vi "Untitled 1.vi"() -> ()   [LabVIEW 2014]
panel:
  out "Waveform Chart 2":dynamicdata(graph)
  in  "Result":dbl
  out "Waveform Chart":dbl(graph)
  in  "Hf":dbl
  out "Elapsed Time (s)":dbl
  in  "H0":dbl
  out "Numeric":dbl
  out "Tank":dbl(slide) scale=0.0..0.3
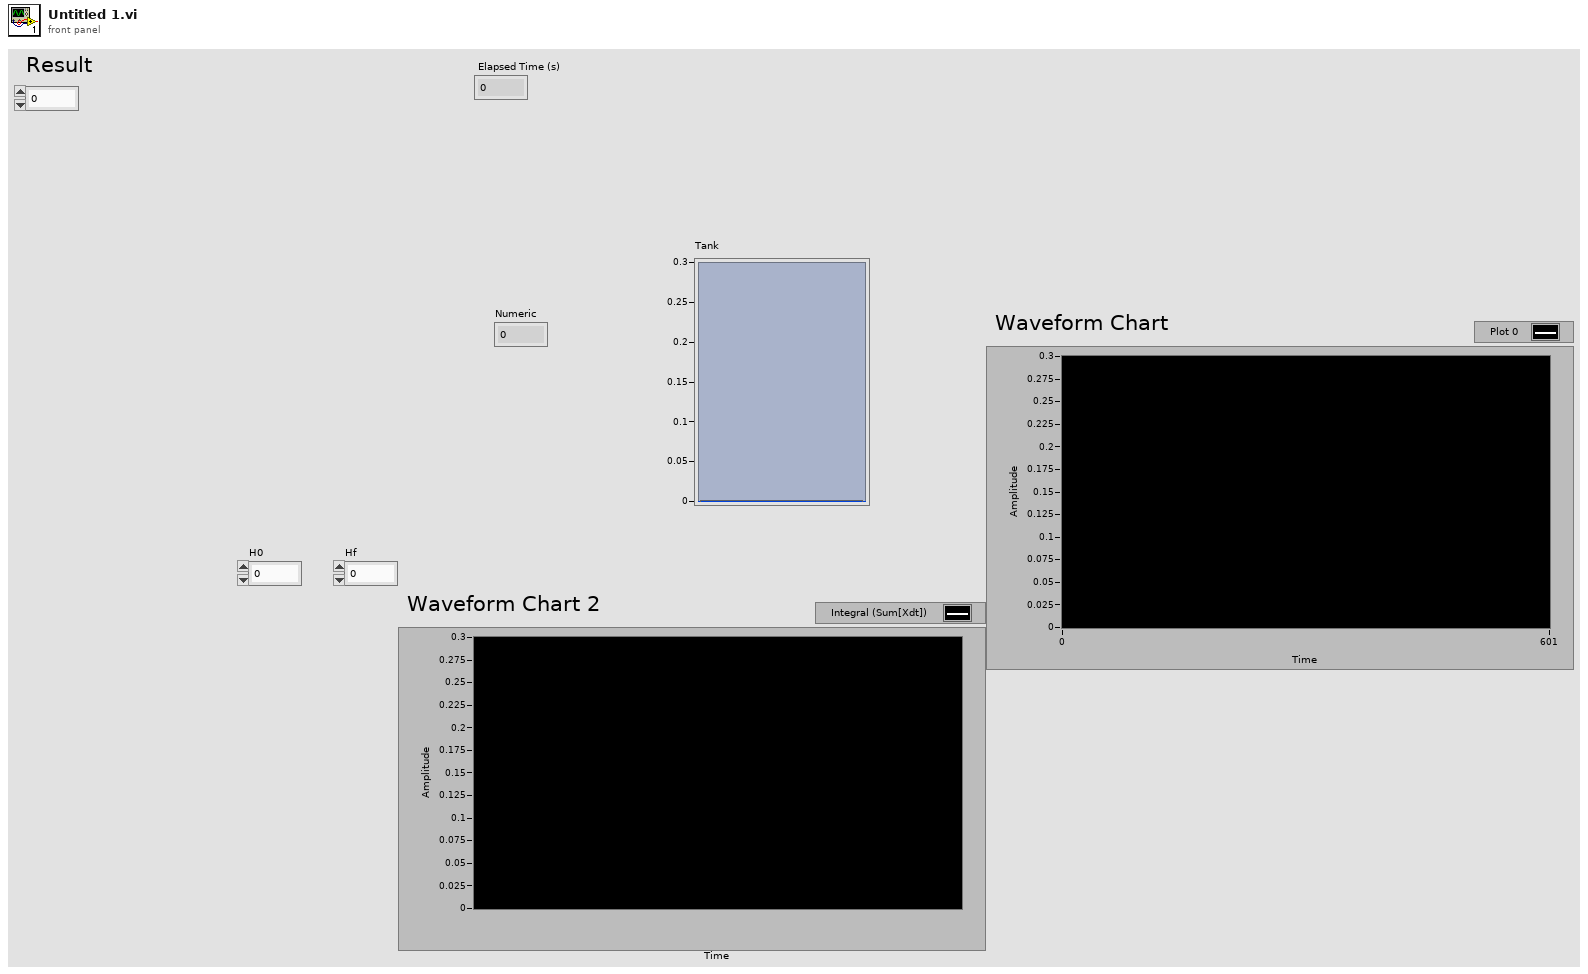
[diagram p1: front panel]
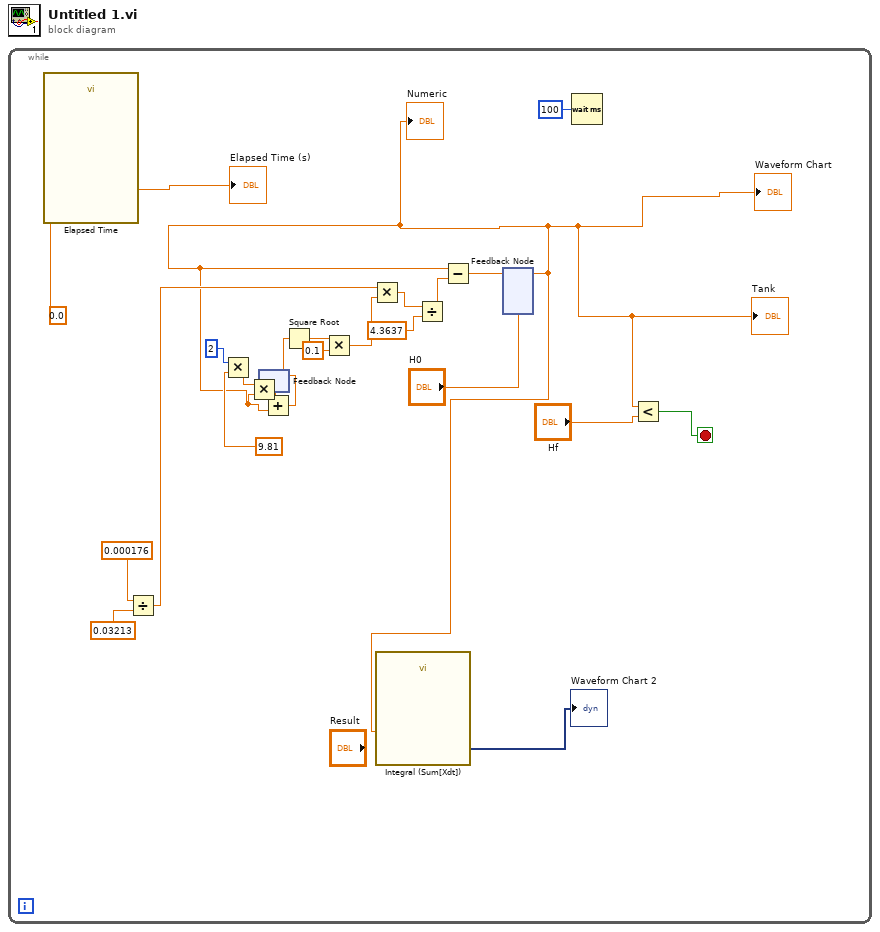
[diagram p0: block diagram]
diagram:
  n1 = while {
    stop <- w8 stop-if-true
    n2 = call "Elapsed Time"("Set Start Time (s)"=0.0) -> ("Elapsed Time (s)"=→"Elapsed Time (s)":dbl)  [unwired: 11 in, 7 out]
    n3 = Divide(x=0.000176 ("A2"), y=0.03213 ("A1")) -> (x/y=w4:dbl)
    n4 = Multiply(x=2, y=9.81 ("G")) -> (x*y=w22:dbl)
    n5 = feedback #1() -> (w19:dbl)  [unwired: 1 in]
    n6 = Square Root(x=w19) -> (sqrt(x)=w15:dbl)
    n7 = Multiply(x=w15, y=0.1) -> (x*y=w13:dbl)
    n8 = Multiply(x=w4, y=w13) -> (x*y=w12:dbl)
    n9 = Divide(x=w12, y=4.3637) -> (x/y=w11:dbl)
    n10 = feedback #2("H0") -> (w2:dbl)
    "Tank" <- w2
    "Numeric" <- w2
    "Waveform Chart" <- w2
    n11 = Multiply(x=w22, y=w2) -> (x*y=w21:dbl)
    n12 = Add(x=w21, y=w2) -> (x+y=w20:dbl)
    n13 = feedback-in #1(w20) -> ()
    n14 = call "Integral (Sum[Xdt])"("Signals"=w2) -> ("Result"=→"Waveform Chart 2":dynamicdata)  [unwired: 5 in, 1 out]
    n15 = Subtract(x=w2, y=w11) -> (x-y=w18:dbl)
    n16 = feedback-in #2(w18) -> ()
    n17 = Wait (ms)(milliseconds to wait=u32 100) -> ()  [unwired: 1 out]
    n18 = Less?(x=w2, y="Hf") -> (x < y?=w8:bool)
  }
